vi "Name and Sort DAT.vi"(4 "Time Stamp Format":string, 5 "Bird Name":string="TEST", 6 "Root Folder":path) -> (1 "Filename":string="TEST_3327427046_2009_06_09_17_17_25.wav", 2 "Append Path":path=path "C:/Users/Bird Brain/Desktop/Audio Recordings/Test Bird/2009-06-09/TEST_3327427046_2009_06_09_17_17_25.wav")   [LabVIEW 2016]
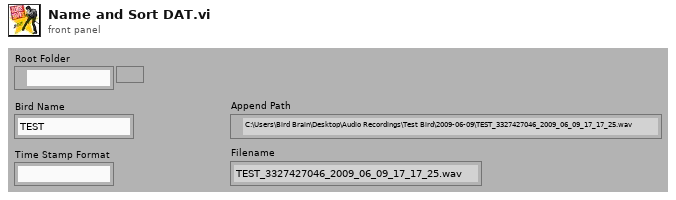
[diagram p1: front panel]
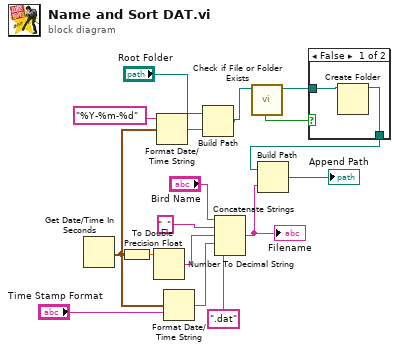
[diagram p0: block diagram]
diagram:
  n1 = Get Date/Time In Seconds() -> (seconds since 1Jan1904=w6:timestamp)
  n2 = To Double Precision Float(number=w6) -> (double precision float=w12:dbl)
  n3 = Number To Decimal String(number=w12) -> (decimal integer string=w10:string)  [unwired: 1 out]
  n4 = Format Date/Time String(time format string (%c)="%Y-%m-%d", seconds (now)=w6) -> (date/time string=w8:string)  [unwired: 1 out]
  n5 = Format Date/Time String(time format string (%c)="Time Stamp Format", seconds (now)=w6) -> (date/time string=w14:string)  [unwired: 1 out]
  n6 = Build Path(base path="Root Folder", name or relative path=w8) -> (appended path=w3:path)
  n7 = Concatenate Strings("Bird Name", "_" ("string"), w10, w14, ".dat" ("string")) -> (w13:string)
  "Filename" <- w13
  n8 = call <vilib>:"Check if File or Folder Exists.vi"("path"=w3) -> ("file or folder exists?"=w4:bool, "dup path"=w5:path)  [unwired: 1 in, 8 out]
  n9 = case shown="False" w4 {
    tunnel: w5 -> [w19 w20]
    tunnel: [w18 w20] -> w17
    frame False {
      n10 = Create Folder(path (use dialog)=w19) -> (created path=w18:path)  [unwired: 1 in, 3 out]
    }
    frame True {
    }
  }
  n11 = Build Path(base path=w17, name or relative path=w13) -> (appended path=→"Append Path":path)
